vi "FindDataFrom2DListCtrl.vi"(9 "column index":u16, 10 "search string":string, 11 "ArrayRef in":refnum<vi>) -> (1 "is empty?":bool, 2 "array out":string[][](array[string]), 3 "ArrayRef out":refnum<vi>)   [LabVIEW 2018, in "Library-Ctrl.lvlib"]
uses:
  Library-Ctrl.lvlib
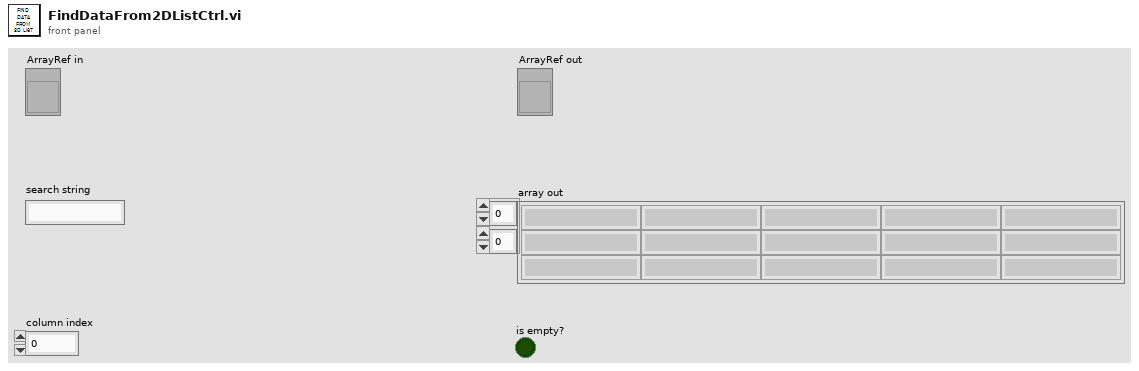
[diagram p1: front panel]
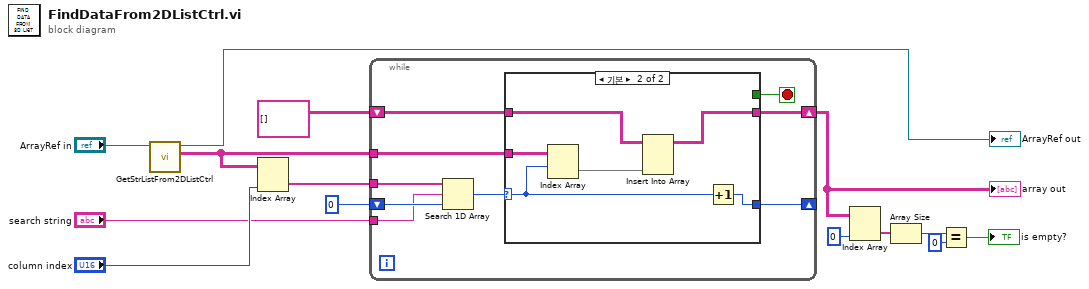
[diagram p0: block diagram]
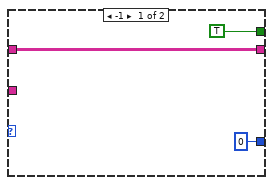
[diagram p2: hidden frame]
diagram:
  n1 = call "GetStrListFrom2DListCtrl.vi"("ref 2D list in"="ArrayRef in") -> ("result"=w7:string[][], "ref 2D list out"=→"ArrayRef out":refnum<vi>)  [unwired: 9 in]
  n2 = Index Array(array=w7, index (col)="column index") -> (element=w11:string[])  [unwired: 1 in]
  n3 = while {
    tunnel: w11 -> [w19]
    shift-right: [w17] -> _
    shift-left: 0 ("시작 인덱스(0)") -> [w23]
    tunnel: "search string" -> [w22]
    shift-right: [w18] -> w6
    shift-left: string[][] [] ("result") -> [w20]
    tunnel: w7 -> [w15]
    stop <- w16 stop-if-true
    n4 = Search 1D Array(1D array=w19, element=w22, start index (0)=w23) -> (index of element=w21:i32)
    n5 = case shown="기본" w21 {
      selector: w21 -> [_ w28]
      tunnel: w20 -> [w26 w32]
      tunnel: [w26 w31] -> w18
      tunnel: [0 w30] -> w17
      tunnel: [TRUE _] -> w16
      tunnel: w15 -> [_ w29]
      frame -1 {
      }
      frame Default {
        n6 = Index Array(array=w29, index (row)=w28) -> (element=w27:string[])  [unwired: 1 in]
        n7 = Insert Into Array(array=w32, new element=w27) -> (w31:string[][])  [unwired: 2 in]
        n8 = Increment(x=w28) -> (x+1=w30:i32)
      }
    }
  }
  "array out" <- w6
  n9 = Index Array(array=w6, index (col)=0 ("비활성화된 인덱스 (열)")) -> (element=w4:string[])  [unwired: 1 in]
  n10 = Array Size(array=w4) -> (size(s)=w3:i32)
  n11 = Equal?(x=w3, y=0) -> (x = y?=→"is empty?":bool)
